vi "File Dialog.vi"   [LabVIEW 2020, in "Reusable Library.lvlib"]
uses:
  <userlib>/_Reusable Library/Reusable Library.lvlib
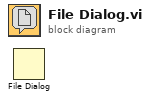
[diagram p0: block diagram]
diagram:
  n1 = File Dialog() -> ()  [unwired: 7 in, 4 out]
